vi "DHE_GetDarkExpTime.vi"() -> (2 "DarkExp":u32)   [LabVIEW 2016]
uses:
  private/vis/DHE_VarAction.ctl
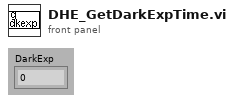
[diagram p1: front panel]
types:
  T1 = typedef "DHE_VarAction.ctl" = enum16{"read", "write"}
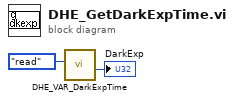
[diagram p0: block diagram]
diagram:
  n1 = call "DHE_VAR_DarkExpTime.vi"("action"=DHE_VarAction."read") -> ("DarkExp"=→"DarkExp":u32)  [unwired: 1 in, 9 out]
